vi "emi_Get Application version.vi"(11 "error in (no error)":errorcluster) -> (4 "Version has been set":bool, 8 "Version Info out":T1={"Name"="Default Name", "Major"=0, "Minor"=0, "Fix"=0, "Build"=0, "Type"=enum."Alfa", "Dev"=FALSE, "Version Name"="", "Date"=timestamp(0 s since 1904-01-01)} {"Date" format="%<%y%m%d>T"}, 15 "error out":errorcluster)   [LabVIEW 2011]
doc: "Set the application version information.\n\nOn error. Sett version anyway, asuming directly from constant."
uses:
  Private/emi_Version Info.ctl
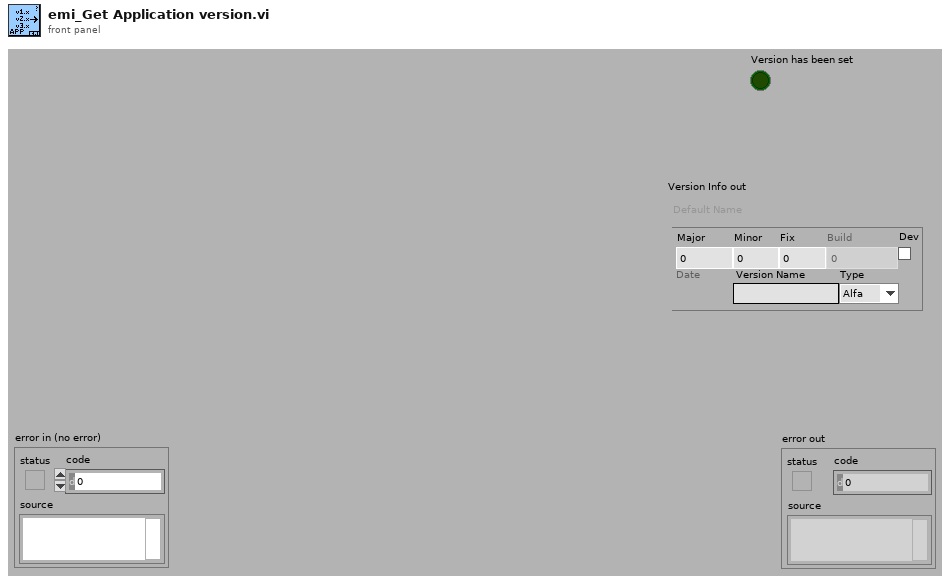
[diagram p1: front panel]
types:
  T1 = typedef "emi_Version Info.ctl" = cluster{"Name":string, "Major":i16, "Minor":i16, "Fix":i16, "Build":i32, "Type":enum16{"Alfa", "Beta", "Stable"}, "Dev":bool, "Version Name":string, "Date":timestamp}
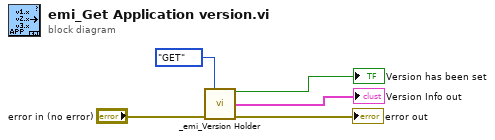
[diagram p0: block diagram]
diagram:
  n1 = call "_emi_Version Holder.vi"("Action(GET)"=enum16{"GET", "SET"}."GET", "error in (no error)"="error in (no error)") -> ("Version set"=→"Version has been set":bool, "Version Info out"=→"Version Info out":T1, "error out"=→"error out":errorcluster)  [unwired: 11 in]
